vi "MainTemplate.vi"() -> ()   [LabVIEW 2017]
uses:
  <vilib>/Utility/cursorutil.llb/Set Cursor (Icon Pict).vi
panel:
  out "Admin?":bool
  out "DAQmx":tag
  in  "EventTimeout":i32=100
  out "TestArray":string[](array[string])
  out "PN":string
  out "FileName":string
  out "UUT SoftwareVer":string
  out "SN From File":string
  out "ProductRev":string
  out "UUT In":u16(ring)=4 items=["BLDC  60A  P/N: 1"=1, "BLDC  30A  P/N: 2"=2, "Warrior 60A P/N: 3"=3, "Condenser Merkava P/N: 4"=4, "Condenser India P/N: 4"=5]
  out "G.Stop":bool
  out "STDBY":bool
  out "TestinExecution":string
  out "User":string
  out "ParamVersion":string
  out "TesterVersion":string
  out "ClosePanel":bool=TRUE
  out "Automation":bool
  out "Test Failed":bool
  out "Next SN":i32
  in  "SetSN":bool
  out "UUT":u8
  out "UUT":string="EBAY"
  in  "Report":bool
  in  "Start":bool
  in  "ATR":string[][](table)=[["Test Communication", "-", "-", "-", "-", ""], ["Set S/N", "-", "-", "-", "-", ""], ["Set Board Number", "-", "-", "-", "-", ""], [" ", "", "", "", "", ""], ["Test Communication", "-", "-", "-", "-", ""], ["Get S/N", "-", "-", "-", "", ""], ["Get Board Number", "-", "-", "-", "", ""], ["Get FW", "-", "-", "-", "", ""], ["Enable Motor", "", "", "", "", ""], ["Small position command", "", "", "", "", ""], ["Measure delta", "", "", "", "", ""], ["Velocity command", "", "", "", "", ""]]
  in  "Settings":bool
  in  "Refresh Button":bool
  in  "VISA":refnum<visa-resource-name>="COM6"
  in  "Help Button":bool
  out "Pannel User Message":string
  in  "Stop Button":bool
  # "Template"
  # "REDLER TECHNOLOGIES LTD"
  # "ver 1.2p"
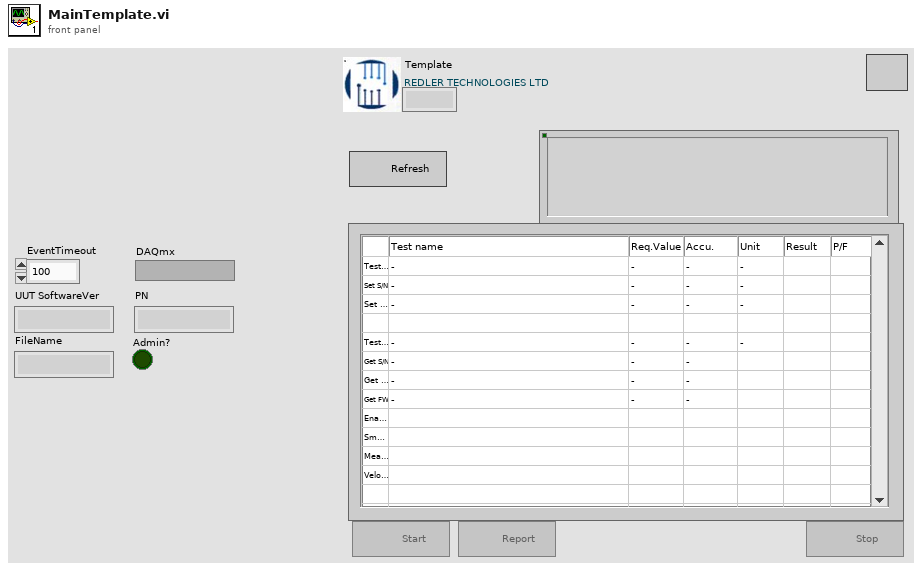
[diagram p1: front panel]
types:
  T1 = cluster{"VISA":refnum<visa-resource-name>, "TestArray":string[]}
  T2 = enum16{"Erase ATR Table", "Stop", "MainProgram", "Initialize"}
  T3 = enum8{"Enabled", "Disabled", "Disabled and Grayed Out"}
  T4 = enum32{"Invalid", "Standard", "Closed", "Hidden", "Minimized", "Maximized"}
  T5 = typedef "LVPoint32TypeDef.ctl" = cluster{"Horizontal":i32, "Vertical":i32}
  T6 = typedef "LVRowAndColumnTypeDef.ctl" = cluster{"Row":i32, "Column":i32}
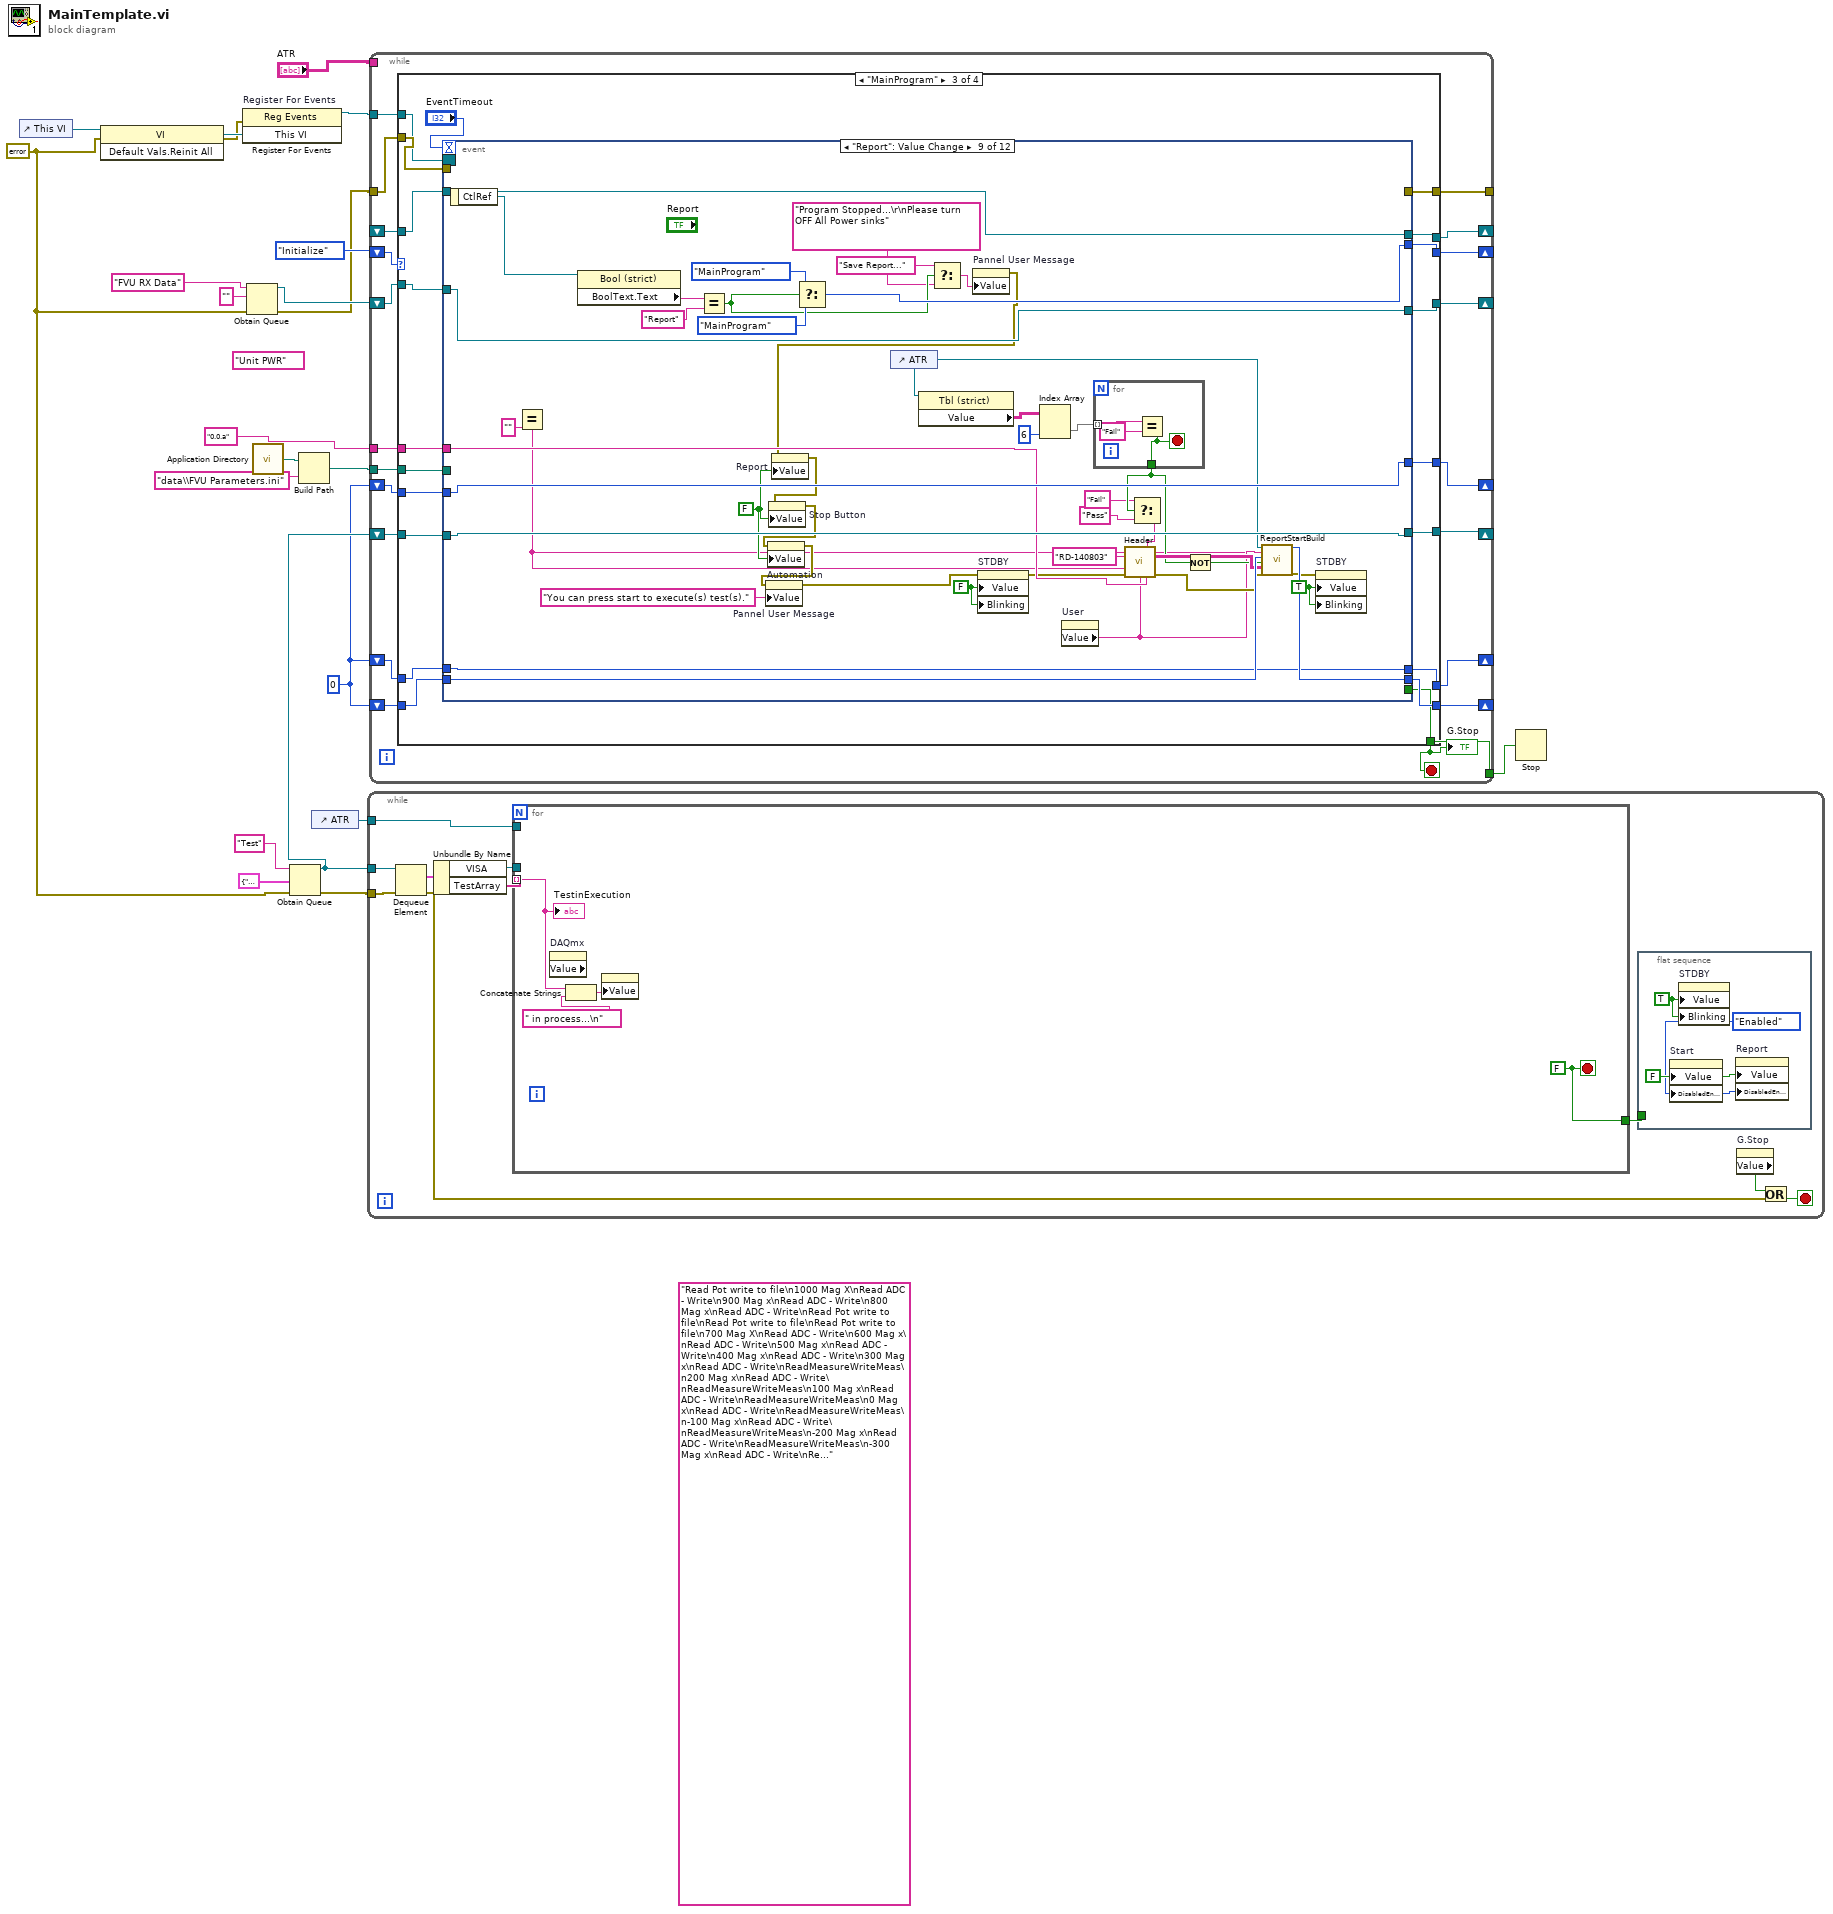
[diagram p0: block diagram]
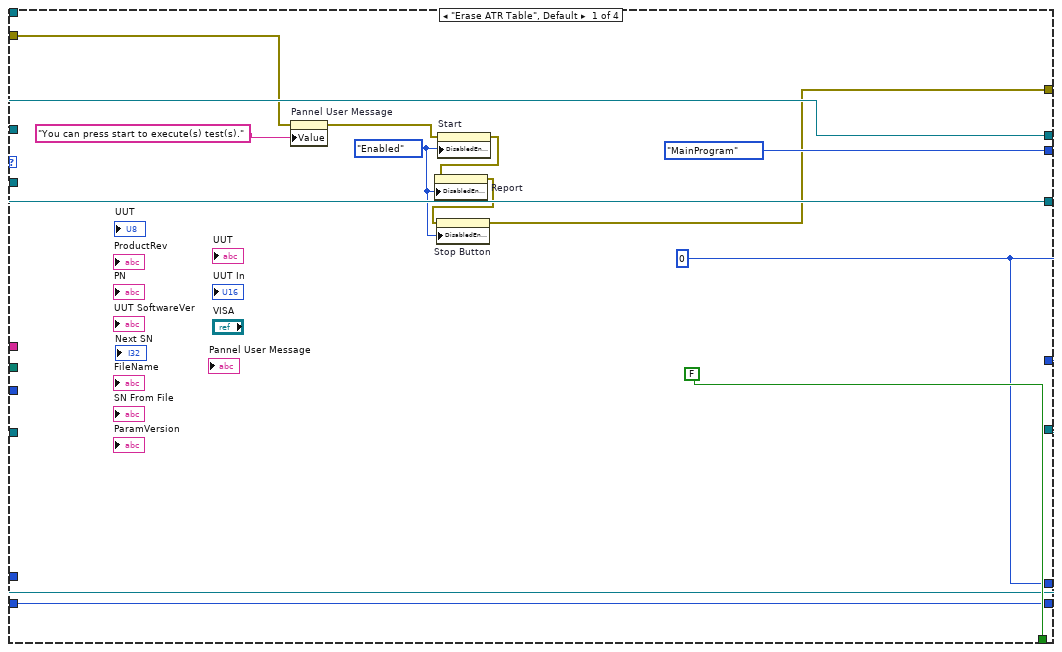
[diagram p2: hidden frame]
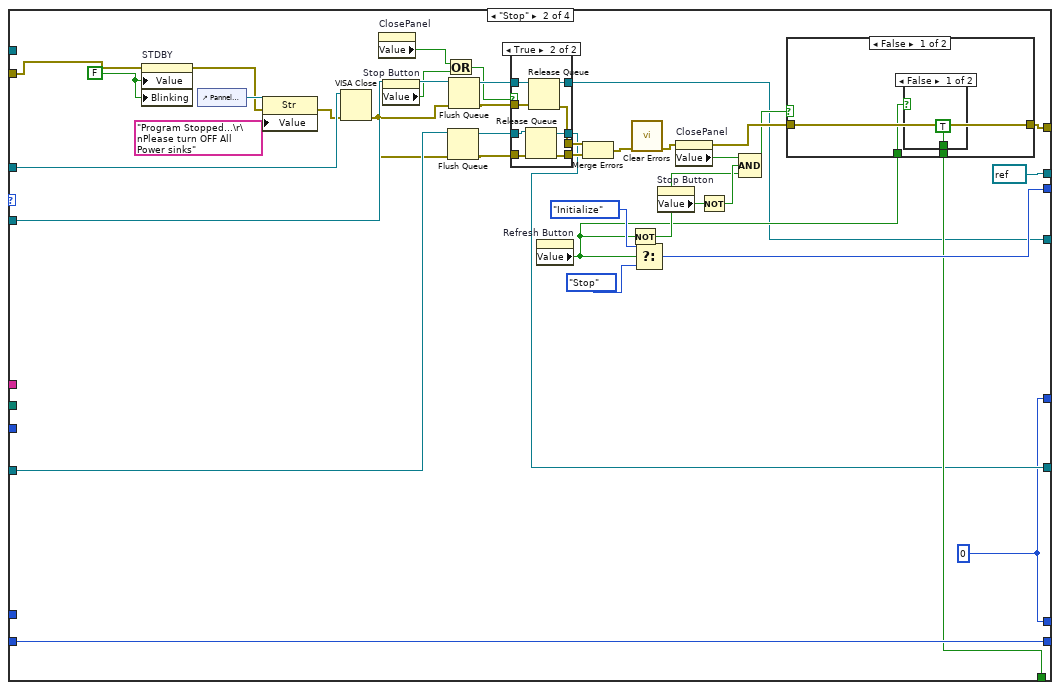
[diagram p3: hidden frame]
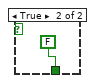
[diagram p5: hidden frame]
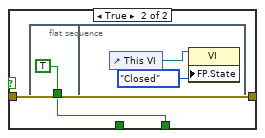
[diagram p6: hidden frame]
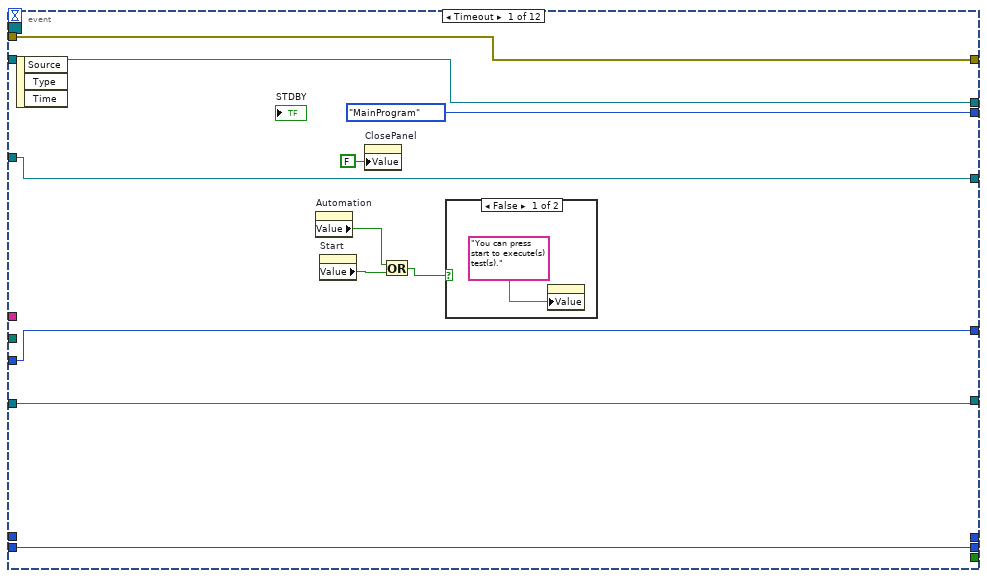
[diagram p7: hidden frame]
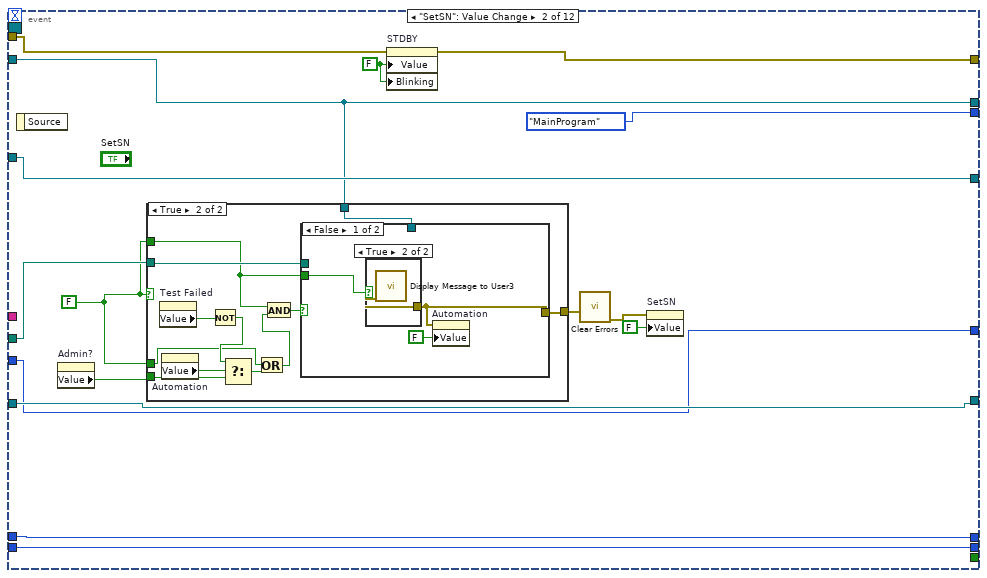
[diagram p9: hidden frame]
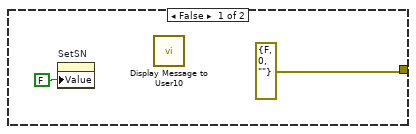
[diagram p10: hidden frame]
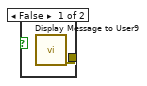
[diagram p11: hidden frame]
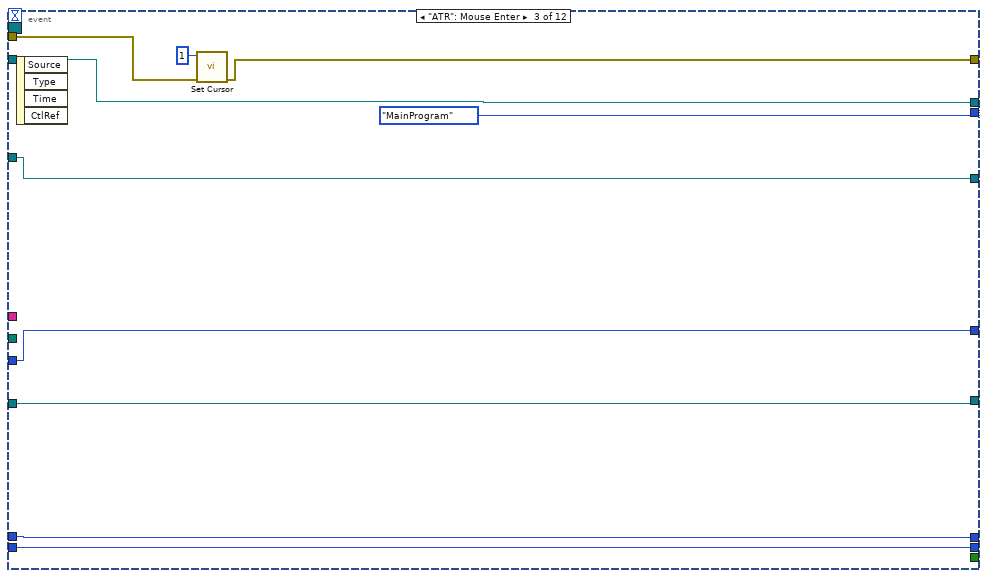
[diagram p13: hidden frame]
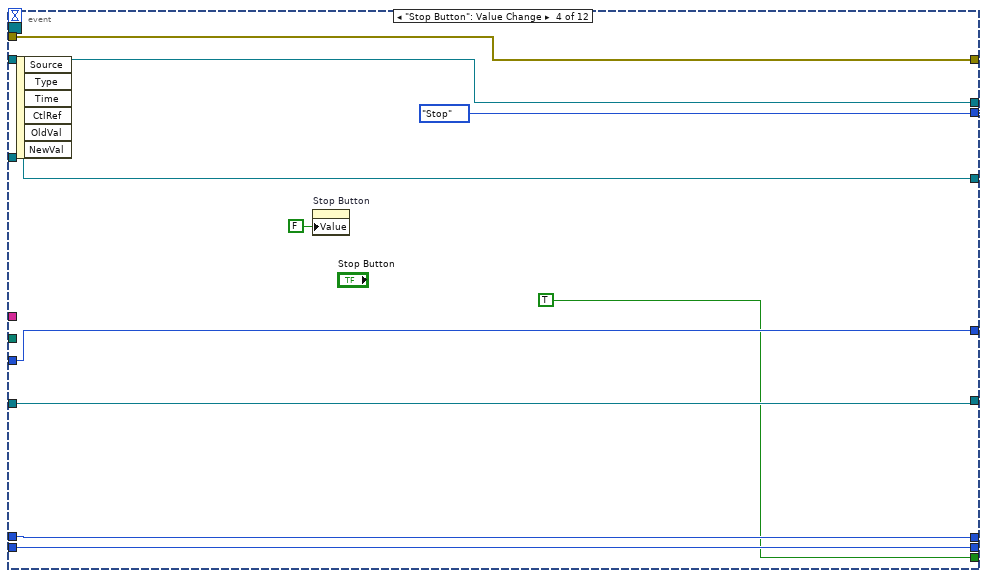
[diagram p14: hidden frame]
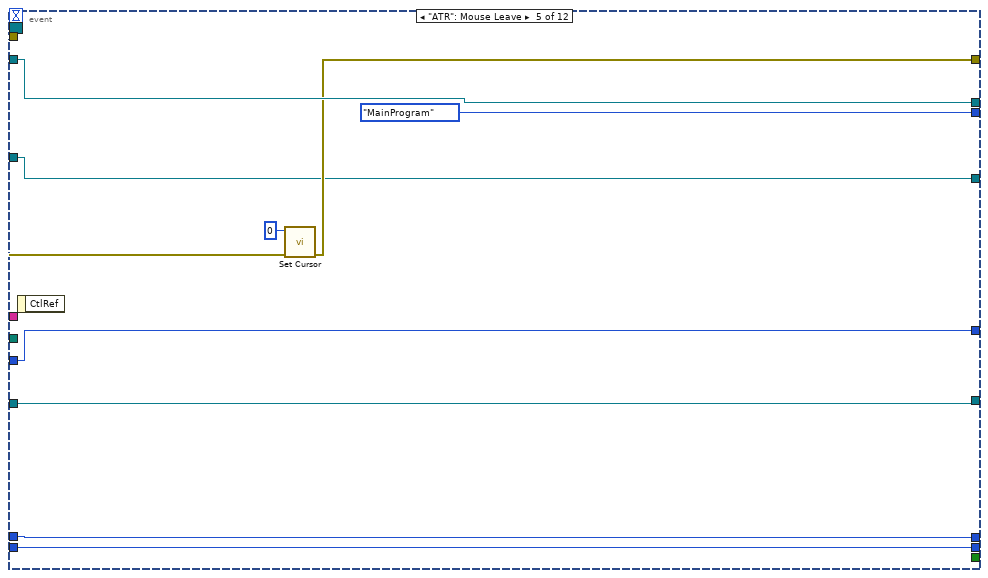
[diagram p15: hidden frame]
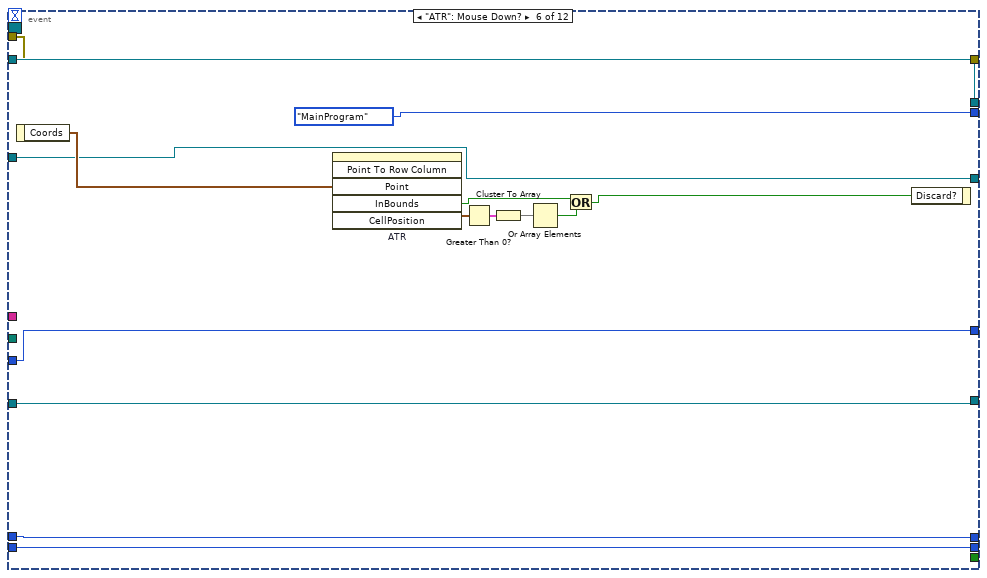
[diagram p16: hidden frame]
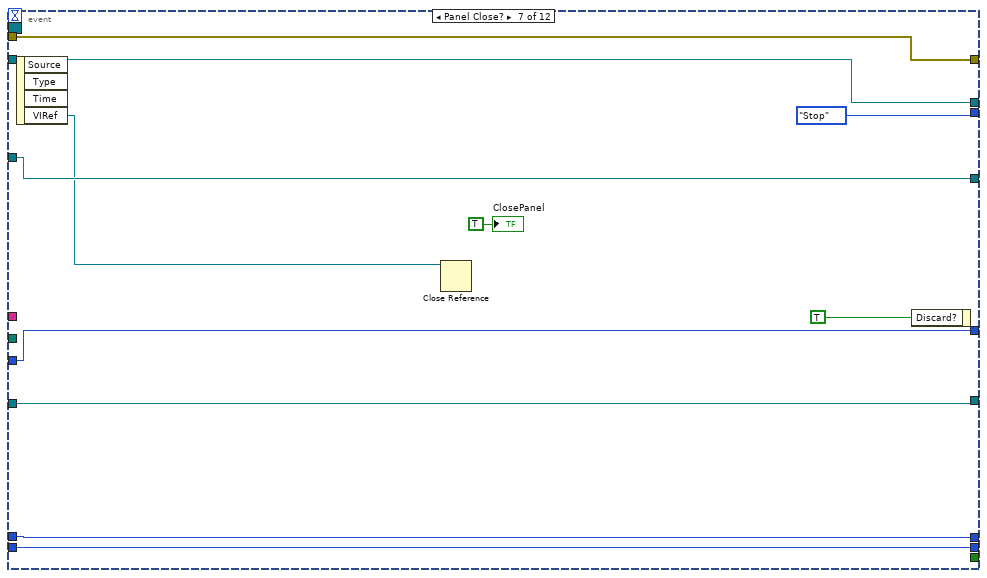
[diagram p17: hidden frame]
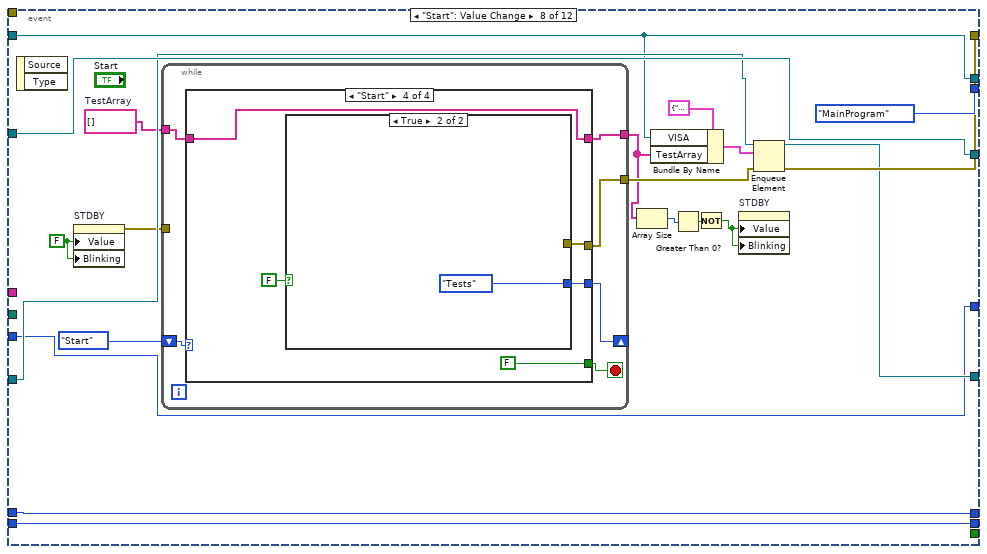
[diagram p18: hidden frame]
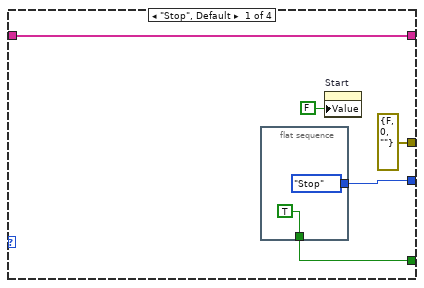
[diagram p19: hidden frame]
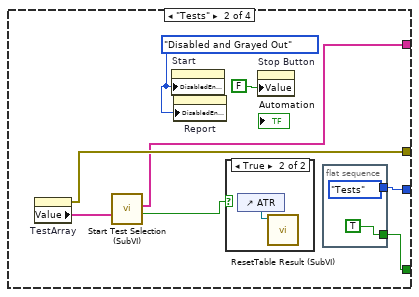
[diagram p20: hidden frame]
diagram:
  (unwired) "Read Pot write to file\n1000 Mag X\nRead ADC - Write\n900 Mag x\nRead ADC - Write\n800 Mag x\nRead ADC - Write\nRead Pot write to file\nRead Pot write to file\nRead Pot write to file\n700 Mag X\nRead ADC - Write\n600 Mag x\nRead ADC - Write\n500 Mag x\nRead ADC - Write\n400 Mag x\nRead ADC - Write\n300 Mag x\nRead ADC - Write\nReadMeasureWriteMeas\n200 Mag x\nRead ADC - Write\nReadMeasureWriteMeas\n100 Mag x\nRead ADC - Write\nReadMeasureWriteMeas\n0 Mag x\nRead ADC - Write\nReadMeasureWriteMeas\n-100 Mag x\nRead ADC - Write\nReadMeasureWriteMeas\n-200 Mag x\nRead ADC - Write\nReadMeasureWriteMeas\n-300 Mag x\nRead ADC - Write\nReadMeasureWriteMeas\n-400 Mag x\nRead ADC - Write\n-500 Mag x\nRead ADC - Write\n-600 Mag x\nRead ADC - Write\nRead Pot write to file\nRead Pot write to file\nRead Pot write to file\n-700 Mag x\nRead ADC - Write\n-800 Mag x\nRead ADC - Write\n-900 Mag x\nRead ADC - Write\n-1000 Mag x\nRead ADC - Write"
  (unwired) "Unit PWR" ("Combo Box")
  w10 = 0
  w3 = errorcluster {"status"=FALSE, "code"=0, "source"=""} ("error in (no error)")
  n1 = control-ref of="This VI"() -> (w11:refnum<vi>)
  n2 = invoke class="VI" method="Default Vals.Reinit All"(reference=w11, error in=w3) -> (reference out=w6:refnum<vi>, error out=w1:errorcluster)  [unwired: 1 in, 1 out]
  n3 = register-events "Register For Events"(error in=w1, w6) -> (reference out=w13:refnum<event-registration>)  [unwired: 1 in, 1 out]
  n4 = Obtain Queue(name (unnamed)="FVU RX Data", element data type="", error in (no error)=w3) -> (queue out=w20:refnum<queue>, error out=w18:errorcluster)  [unwired: 2 in, 1 out]
  n5 = call <vilib>:"Application Directory.vi"() -> ("Application Directory"=w15:path)
  n6 = Obtain Queue(name (unnamed)="Test", element data type=T1 {"VISA"="COM1", "TestArray"=[]}, error in (no error)=w3) -> (queue out=w17:refnum<queue>, error out=w2:errorcluster)  [unwired: 2 in, 1 out]
  n7 = Build Path(base path=w15, name or relative path="data\\FVU Parameters.ini") -> (appended path=w7:path)
  n8 = control-ref of="ATR"() -> (w12:refnum<vi>)
  n9 = while {
    tunnel: w12 -> [w32]
    tunnel: w2 -> [w30]
    tunnel: w17 -> [w31]
    stop <- w24 stop-if-true
    n10 = Dequeue Element(queue=w31, error in (no error)=w30) -> (element=w29:T1, error out=w27:errorcluster)  [unwired: 1 in, 2 out]
    n11 = Unbundle By Name(w29) -> ("VISA"=w28:refnum<visa-resource-name>, "TestArray"=w25:string[])
    n12 = for {
      tunnel: w25 -> [w37] mode=indexing
      tunnel: w28 -> [_]
      tunnel: w32 -> [_]
      tunnel: [w39] -> w26
      stop <- w39 stop-if-true
      w39 = FALSE ("Stopped")
      n13 = property on="DAQmx" class="DAQmxName" props=["Value"]() -> ()  [unwired: 2 in, 3 out]
      n14 = Concatenate Strings(w37, " in process...\n" ("string")) -> (w36:string)
      n15 = property on="Pannel User Message" class="Str"("Value"=w36) -> ()  [unwired: 2 in, 2 out]
      "TestinExecution" <- w37
    }
    n16 = flat-sequence {
      tunnel: w26 -> [_]
      frame #0 {
        w33 = TRUE ("STDBY")
        w34 = T3."Enabled" ("Disabled")
        w35 = FALSE ("Start")
        n17 = property on="Start" class="Bool (strict)"("Value"=w35, "DisabledEnum"=w34) -> ()  [unwired: 2 in, 2 out]
        n18 = property on="STDBY" class="Bool (strict)"("Value"=w33, "Blinking"=w33) -> ()  [unwired: 2 in, 2 out]
        n19 = property on="Report" class="Bool (strict)"("Value"=w35, "DisabledEnum"=w34) -> ()  [unwired: 2 in, 2 out]
      }
    }
    n20 = property on="G.Stop" class="Bool (strict)"() -> ("Value"=w23:bool)  [unwired: 2 in, 2 out]
    n21 = Or(x=w23, y=w27) -> (x .or. y?=w24:bool)
  }
  n22 = while {
    shift-right: [w46] -> _
    shift-left: T2."Initialize" -> [w40]
    shift-right: [w57] -> _
    shift-left: _ -> [w56]
    shift-right: [w55] -> _
    shift-left: w20 -> [w54]
    shift-right: [w52] -> _
    shift-left: w17 -> [w53]
    tunnel: "ATR" -> [_]
    tunnel: w13 -> [w51]
    shift-right: [w49] -> _
    shift-left: w10 -> [w50]
    tunnel: w7 -> [w48]
    tunnel: w18 -> [w59]
    tunnel: [w58] -> _
    tunnel: "0.0.a" -> [w47]
    shift-right: [w44] -> _
    shift-left: w10 -> [w45]
    shift-right: [w42] -> _
    shift-left: w10 -> [w43]
    tunnel: [w41] -> w8
    stop <- w41 stop-if-true
    n23 = case shown="\"MainProgram\"" w40 {
      tunnel: [T2."MainProgram" w98 w151 T2."Erase ATR Table"] -> w46
      tunnel: [FALSE w87 w132 FALSE] -> w41
      tunnel: [w61 w91 w146 w395] -> w58
      tunnel: w59 -> [w60 w78 w150 w395]
      tunnel: [w63 refnum<visa-resource-name> refnum ("VISA resource name") w147 w392] -> w57
      tunnel: w56 -> [w63 w108 w148 _]
      tunnel: [w72 w81 w144 w398] -> w55
      tunnel: w54 -> [w72 w110 w145 w398]
      tunnel: w53 -> [w71 w104 w143 w397]
      tunnel: [w71 w80 w142 w397] -> w52
      tunnel: w51 -> [_ _ w141 _]
      tunnel: w50 -> [w70 w102 w140 w396]
      tunnel: [w70 w102 w139 w396] -> w49
      tunnel: w48 -> [_ _ w138 _]
      tunnel: w47 -> [_ _ w137 w391]
      tunnel: w45 -> [_ _ w136 _]
      tunnel: [w69 w79 w135 w394] -> w44
      tunnel: w43 -> [_ _ w134 _]
      tunnel: [w69 w79 w133 w394] -> w42
      frame "Erase ATR Table", Default {
        w69 = 0
        w64 = T3."Enabled" ("Disabled")
        n24 = property on="Pannel User Message" class="Str"(error in=w60, "Value"="You can press start to execute(s) test(s)." ("Pannel User Message")) -> (error out=w62:errorcluster)  [unwired: 1 in, 1 out]
        n25 = property on="Start" class="Bool (strict)"(error in=w62, "DisabledEnum"=w64) -> (error out=w67:errorcluster)  [unwired: 1 in, 1 out]
        n26 = property on="Report" class="Bool (strict)"(error in=w67, "DisabledEnum"=w64) -> (error out=w65:errorcluster)  [unwired: 1 in, 1 out]
        n27 = property on="Stop Button" class="Bool (strict)"(error in=w65, "DisabledEnum"=w64) -> (error out=w61:errorcluster)  [unwired: 1 in, 1 out]
      }
      frame "Stop" {
        w77 = FALSE ("STDBY")
        w79 = 0
        n28 = property on="STDBY" class="Bool (strict)"(error in=w78, "Value"=w77, "Blinking"=w77) -> (error out=w74:errorcluster)  [unwired: 1 in, 1 out]
        n29 = control-ref of="Pannel User Message"() -> (w76:refnum<vi>)
        n30 = property class="Str"(reference=w76, error in=w74, "Value"="Program Stopped...\r\nPlease turn OFF All Power sinks") -> (error out=w101:errorcluster)  [unwired: 1 out]
        n31 = VISA Close(VISA resource name=w108, error in (no error)=w101) -> (error out=w103:errorcluster)
        n32 = property on="ClosePanel" class="Bool (strict)"() -> ("Value"=w84:bool)  [unwired: 2 in, 2 out]
        n33 = property on="Stop Button" class="Bool (strict)"() -> ("Value"=w83:bool)  [unwired: 2 in, 2 out]
        n34 = Or(x=w84, y=w83) -> (x .or. y?=w82:bool)
        n35 = Flush Queue(queue=w104, error in (no error)=w103) -> (queue out=w106:refnum<queue>, error out=w105:errorcluster)  [unwired: 1 out]
        n36 = Flush Queue(queue=w110, error in (no error)=w103) -> (queue out=w109:refnum<queue>, error out=w111:errorcluster)  [unwired: 1 out]
        n37 = case shown="True" w82 {
          tunnel: w111 -> [w113 w121]
          tunnel: w109 -> [w115 w117]
          tunnel: w106 -> [w114 w116]
          tunnel: w105 -> [w112 w120]
          tunnel: [w113 w119] -> w97
          tunnel: [w112 w118] -> w96
          tunnel: [w115 w117] -> w81
          tunnel: [w114 w116] -> w80
          frame False {
          }
          frame True {
            n38 = Release Queue(queue=w116, error in (no error)=w120) -> (error out=w118:errorcluster)  [unwired: 1 in, 2 out]
            n39 = Release Queue(queue=w117, error in (no error)=w121) -> (error out=w119:errorcluster)  [unwired: 1 in, 2 out]
          }
        }
        n40 = property on="Refresh Button" class="Bool (strict)"() -> ("Value"=w85:bool)  [unwired: 2 in, 2 out]
        n41 = Merge Errors(w97, w96) -> (w95:errorcluster)
        n42 = Not(x=w85) -> (.not. x?=w86:bool)
        n43 = call <vilib>:"Clear Errors.vi"("error in (no error)"=w95) -> ("error out"=w94:errorcluster)  [unwired: 5 in, 1 out]
        n44 = Select(t=T2."Initialize", s=w85, f=T2."Stop") -> (s? t:f=w98:T2)
        n45 = property on="Stop Button" class="Bool (strict)"() -> ("Value"=w89:bool)  [unwired: 2 in, 2 out]
        n46 = property on="ClosePanel" class="Bool (strict)"(error in=w94) -> (error out=w92:errorcluster, "Value"=w93:bool)  [unwired: 1 in, 1 out]
        n47 = Not(x=w89) -> (.not. x?=w88:bool)
        n48 = Compound Arithmetic op=AND(w93, w88, w86) -> (w90:bool)
        n49 = case shown="False" w90 {
          tunnel: w92 -> [w124 w128]
          tunnel: [w124 w128] -> w91
          tunnel: [w123 w127] -> w87
          tunnel: w85 -> [w122 _]
          frame False {
            n50 = case shown="False" w122 {
              tunnel: [TRUE FALSE] -> w123
              frame False {
              }
              frame True {
              }
            }
          }
          frame True {
            n51 = flat-sequence {
              tunnel: [TRUE] -> w127
              frame #0 {
              }
              frame #1 {
                n52 = control-ref of="This VI"() -> (w131:refnum<vi>)
                n53 = property class="VI"(reference=w131, "FP.State"=T4."Closed" ("Front Panel Window:State")) -> ()  [unwired: 1 in, 2 out]
              }
            }
          }
        }
      }
      frame "MainProgram" {
        n54 = event shown="[8] \"Report\": Value Change" {
          selector: w141 -> [_ _ _ _ _ _ _ _ _ _ _ _]
          dyn-events: _ -> [_ _ _ _ _ _ _ _ _ _ _ _]
          timeout: "EventTimeout" -> [_ _ _ _ _ _ _ _ _ _ _ _]
          tunnel: [T2."MainProgram" T2."MainProgram" T2."MainProgram" T2."Stop" T2."MainProgram" T2."MainProgram" T2."Stop" T2."MainProgram" w346 T2."MainProgram" T2."Stop" T2."MainProgram"] -> w151
          tunnel: [w158 w165 w207 w217 w225 w235 w254 w271 w339 w370 w382 w383] -> w146
          tunnel: w150 -> [w158 w168 w206 w217 w227 w235 w254 _ w339 w359 w382 w383]
          tunnel: [w156 w174 w208 w218 w226 w236 w252 w264 w312 w368 w380 w386] -> w147
          tunnel: w148 -> [w156 w174 w208 w218 w226 w236 w252 w264 w312 w368 w380 w386]
          tunnel: w145 -> [w161 w179 w203 w215 w223 w233 w251 w273 w354 w367 w379 w389]
          tunnel: [w161 w179 w203 w215 w223 w233 w251 w273 w354 w367 w379 w389] -> w144
          tunnel: w143 -> [w155 w178 w202 w214 w222 w232 w250 w272 w353 w366 w378 w388]
          tunnel: [w155 w178 w202 w214 w222 w232 w250 w270 w353 w366 w378 w388] -> w142
          tunnel: w140 -> [w160 w177 w201 w213 w221 w231 w248 w268 w352 w365 w377 w387]
          tunnel: [w160 w177 w201 w213 w221 w231 w248 w268 w351 w365 w377 w387] -> w139
          tunnel: w138 -> [_ w175 _ _ _ _ _ _ _ _ _ _]
          tunnel: w137 -> [_ _ _ _ _ _ _ _ w333 w364 _ _]
          tunnel: w136 -> [_ w170 w200 w212 w220 w230 w245 w267 w340 w362 w376 w385]
          tunnel: [_ w170 w200 w212 w220 w230 w245 w267 w340 w362 w376 w385] -> w135
          tunnel: w134 -> [w157 w169 w199 w211 w219 w229 w244 w266 w337 w361 w375 w384]
          tunnel: [w157 w169 w199 w211 w219 w229 w244 w266 w337 w361 w375 w384] -> w133
          tunnel: [_ _ _ TRUE _ _ _ _ _ _ _ _] -> w132
          event Timeout {
            n55 = event-data() -> ()  [unwired: 1 in, 3 out]
            n56 = property on="Automation" class="Bool (strict)"() -> ("Value"=w154:bool)  [unwired: 2 in, 2 out]
            n57 = property on="Start" class="Bool (strict)"() -> ("Value"=w152:bool)  [unwired: 2 in, 2 out]
            n58 = property on="ClosePanel" class="Bool (strict)"("Value"=FALSE ("ClosePanel")) -> ()  [unwired: 2 in, 2 out]
            n59 = Or(x=w154, y=w152) -> (x .or. y?=w153:bool)
            n60 = case shown="False" w153 {
              frame False {
                n61 = property on="Pannel User Message" class="Str"("Value"="You can press start to execute(s) test(s).") -> ()  [unwired: 2 in, 2 out]
              }
              frame True {
              }
            }
          }
          event "SetSN": Value Change {
            w164 = FALSE ("Value")
            w167 = FALSE ("STDBY")
            n62 = event-data() -> ()  [unwired: 1 in, 1 out]
            n63 = property on="Admin?" class="Bool (strict)"() -> ("Value"=w166:bool)  [unwired: 2 in, 2 out]
            n64 = case shown="True" w164 {
              tunnel: w175 -> [_ w193]
              tunnel: w164 -> [_ w182]
              tunnel: w174 -> [_ w192]
              tunnel: w166 -> [_ w191]
              tunnel: [errorcluster {"status"=FALSE, "code"=0, "source"=""} ("error out") w190] -> w173
              tunnel: w164 -> [_ w183]
              frame False {
                n65 = property on="SetSN" class="Bool (strict)"("Value"=FALSE) -> ()  [unwired: 2 in, 2 out]
                n66 = call "Display Message to User10"() -> ()  [unwired: 10 in, 2 out]
              }
              frame True {
                n67 = property on="Test Failed" class="Bool (strict)"() -> ("Value"=w187:bool)  [unwired: 2 in, 2 out]
                n68 = property on="Automation" class="Bool (strict)"() -> ("Value"=w189:bool)  [unwired: 2 in, 2 out]
                n69 = Not(x=w187) -> (.not. x?=w188:bool)
                n70 = Select(t=w188, s=w189, f=w191) -> (s? t:f=w185:bool)
                n71 = Or(x=w183, y=w185) -> (x .or. y?=w184:bool)
                n72 = And(x=w182, y=w184) -> (x .and. y?=w186:bool)
                n73 = case shown="False" w186 {
                  tunnel: w193 -> [_ _]
                  tunnel: w192 -> [_ _]
                  tunnel: [w195 _] -> w190
                  tunnel: w182 -> [w194 _]
                  frame False {
                    n74 = case shown="True" w194 {
                      tunnel: [w197 w198] -> w195
                      frame False {
                        n75 = call "Display Message to User9"() -> ("error out"=w197:errorcluster)  [unwired: 10 in, 1 out]
                      }
                      frame True {
                        n76 = call "Display Message to User3"() -> ("error out"=w198:errorcluster)  [unwired: 10 in, 1 out]
                      }
                    }
                    n77 = property on="Automation" class="Bool (strict)"(error in=w195, "Value"=FALSE ("Automation")) -> ()  [unwired: 1 in, 2 out]
                  }
                  frame True {
                  }
                }
              }
            }
            n78 = property on="STDBY" class="Bool (strict)"(error in=w168, "Value"=w167, "Blinking"=w167) -> (error out=w165:errorcluster)  [unwired: 1 in, 1 out]
            n79 = call <vilib>:"Clear Errors.vi"("error in (no error)"=w173) -> ("error out"=w171:errorcluster)  [unwired: 5 in, 1 out]
            n80 = property on="SetSN" class="Bool (strict)"(error in=w171, "Value"=FALSE ("SetSN")) -> ()  [unwired: 1 in, 2 out]
          }
          event "ATR": Mouse Enter {
            n81 = event-data() -> ()  [unwired: 1 in, 4 out]
            n82 = call-poly <vilib>:"Set Cursor.vi"("error in (no error)"=w206, "icon"=u16 1) -> ("error out"=w207:errorcluster)  [unwired: 8 in, 1 out]
          }
          event "Stop Button": Value Change {
            n83 = event-data() -> ()  [unwired: 1 in, 6 out]
            n84 = property on="Stop Button" class="Bool (strict)"("Value"=FALSE ("Stop Button")) -> ()  [unwired: 2 in, 2 out]
          }
          event "ATR": Mouse Leave {
            n85 = event-data() -> ()  [unwired: 1 in, 1 out]
            n86 = call-poly <vilib>:"Set Cursor.vi"("error in (no error)"=w227, "icon"=u16 0) -> ("error out"=w225:errorcluster)  [unwired: 8 in, 1 out]
          }
          event "ATR": Mouse Down? {
            n87 = event-data() -> ("Coords"=w243:T5)  [unwired: 1 in]
            n88 = invoke on="ATR" class="Tbl (strict)" method="Point To Row Column"("Point"=w243) -> ("InBounds"=w239:bool, "CellPosition"=w238:T6)  [unwired: 5 in, 4 out]
            n89 = Greater Than 0?(x=w238) -> (x > 0?=w242:cluster{"Row":bool, "Column":bool})
            n90 = Cluster To Array(cluster=w242) -> (array=w241:bool[])
            n91 = Or Array Elements(Boolean array=w241) -> (logical OR=w240:bool)
            n92 = Or(x=w239, y=w240) -> (x .or. y?=w237:bool)
            n93 = event-data("Discard?"=w237) -> ()  [unwired: 1 in, 1 out]
          }
          event Panel Close? {
            n94 = event-data() -> ("VIRef"=w249:refnum<vi>)  [unwired: 1 in, 3 out]
            n95 = Close Reference(reference=w249) -> ()  [unwired: 1 in, 1 out]
            n96 = event-data("Discard?"=TRUE) -> ()  [unwired: 1 in, 1 out]
            "ClosePanel" <- TRUE ("ClosePanel")
          }
          event "Start": Value Change {
            w260 = FALSE ("STDBY")
            w262 = string[] []  # TestArray
            n97 = event-data() -> ()  [unwired: 1 in, 2 out]
            n98 = property on="STDBY" class="Bool (strict)"("Value"=w260, "Blinking"=w260) -> (error out=w261:errorcluster)  [unwired: 2 in, 1 out]
            n99 = while {
              tunnel: [w280] -> w258
              tunnel: [w279] -> w259
              shift-right: [w277] -> _
              shift-left: enum16{"Stop", "Tests", "Bit test", "Start"}."Start" -> [w278]
              tunnel: w262 -> [w276]
              tunnel: w261 -> [_]
              stop <- w275 stop-if-true
              n100 = case shown="\"Start\"" w278 {
                tunnel: [w285 w288 w299 w307] -> w280
                tunnel: [errorcluster {"status"=FALSE, "code"=0, "source"=""} ("error out") w291 errorcluster {"status"=FALSE, "code"=0, "source"=""} ("error out") w305] -> w279
                tunnel: [w284 w295 enum16{"Stop", "Tests", "Bit test", "Start"}."Stop" w304] -> w277
                tunnel: w276 -> [w285 _ w299 w307]
                tunnel: [w283 w294 FALSE FALSE] -> w275
                frame "Stop", Default {
                  n101 = flat-sequence {
                    tunnel: [enum16{"Stop", "Tests", "Bit test", "Start"}."Stop"] -> w284
                    tunnel: [TRUE] -> w283
                    frame #0 {
                    }
                  }
                  n102 = property on="Start" class="Bool (strict)"("Value"=FALSE ("Start")) -> ()  [unwired: 2 in, 2 out]
                }
                frame "Tests" {
                  w293 = T3."Disabled and Grayed Out" ("Disabled")
                  n103 = property on="TestArray" class="Arr (strict)"() -> (error out=w291:errorcluster, "Value"=w290:string[])  [unwired: 2 in, 1 out]
                  n104 = call "Start Test Selection (SubVI).vi"("TestArrayIn"=w290) -> ("AutoOut"=w289:bool, "TestArrayOut"=w288:string[])  [unwired: 9 in]
                  n105 = property on="Start" class="Bool (strict)"("DisabledEnum"=w293) -> ()  [unwired: 2 in, 2 out]
                  n106 = property on="Report" class="Bool (strict)"("DisabledEnum"=w293) -> ()  [unwired: 2 in, 2 out]
                  n107 = case shown="True" w289 {
                    frame False {
                    }
                    frame True {
                      n108 = control-ref of="ATR"() -> (w296:refnum<vi>)
                      n109 = call "ResetTable Result (SubVI).vi"("Table in"=w296) -> ()  [unwired: 11 in]
                    }
                  }
                  n110 = property on="Stop Button" class="Bool (strict)"("Value"=FALSE ("Stop Burn-in")) -> ()  [unwired: 2 in, 2 out]
                  n111 = flat-sequence {
                    tunnel: [enum16{"Stop", "Tests", "Bit test", "Start"}."Tests"] -> w295
                    tunnel: [TRUE] -> w294
                    frame #0 {
                    }
                  }
                }
                frame "Bit test" {
                }
                frame "Start" {
                  n112 = case shown="True" FALSE {
                    tunnel: [w309 _] -> w305
                    tunnel: [enum16{"Stop", "Tests", "Bit test", "Start"}."Stop" enum16{"Stop", "Tests", "Bit test", "Start"}."Tests"] -> w304
                    frame False {
                      n113 = call "Display Message to User5"() -> ("error out"=w309:errorcluster)  [unwired: 10 in, 1 out]
                    }
                    frame True {
                    }
                  }
                }
              }
            }
            n114 = Array Size(array=w258) -> (size(s)=w257:i32)
            n115 = Bundle By Name(cluster=T1 {"VISA"="COM1", "TestArray"=[]}, "VISA"=w264, "TestArray"=w258) -> (w265:T1)
            n116 = Greater Than 0?(x=w257) -> (x > 0?=w256:bool)
            n117 = Not(x=w256) -> (.not. x?=w255:bool)
            n118 = property on="STDBY" class="Bool (strict)"("Value"=w255, "Blinking"=w255) -> ()  [unwired: 2 in, 2 out]
            n119 = Enqueue Element(queue=w272, element=w265, error in (no error)=w259) -> (queue out=w270:refnum<queue>, error out=w271:errorcluster)  [unwired: 2 out]
          }
          event "Report": Value Change {
            w311 = ""
            w316 = FALSE ("Report")
            w335 = TRUE ("STDBY")
            w338 = FALSE ("STDBY")
            n120 = event-data() -> ("CtlRef"=w350:refnum<vi>)  [unwired: 1 in]
            n121 = Equal?(x=w311, y=w311) -> ()  [unwired: 1 out]
            n122 = property class="Bool (strict)"(reference=w350) -> ("BoolText.Text"=w349:string)  [unwired: 1 in, 2 out]
            n123 = Equal?(x=w349, y="Report") -> (x = y?=w344:bool)
            n124 = Select(t=T2."MainProgram", s=w344, f=T2."MainProgram") -> (s? t:f=w346:T2)
            n125 = control-ref of="ATR"() -> (w331:refnum<vi>)
            n126 = property class="Tbl (strict)"(reference=w331) -> ("Value"=w330:string[][])  [unwired: 1 in, 2 out]
            n127 = Select(t="Save Report...", s=w344, f="Program Stopped...\r\nPlease turn OFF All Power sinks") -> (s? t:f=w342:string)
            n128 = property on="Pannel User Message" class="Str"("Value"=w342) -> (error out=w313:errorcluster)  [unwired: 2 in, 1 out]
            n129 = property on="Report" class="Bool (strict)"(error in=w313, "Value"=w316) -> (error out=w319:errorcluster)  [unwired: 1 in, 1 out]
            n130 = property on="Stop Button" class="Bool (strict)"(error in=w319, "Value"=w316) -> (error out=w318:errorcluster)  [unwired: 1 in, 1 out]
            n131 = property on="Automation" class="Bool (strict)"(error in=w318, "Value"=w316) -> (error out=w317:errorcluster)  [unwired: 1 in, 1 out]
            n132 = property on="Pannel User Message" class="Str"(error in=w317, "Value"="You can press start to execute(s) test(s)." ("Pannel User Message")) -> (error out=w314:errorcluster)  [unwired: 1 in, 1 out]
            n133 = property on="STDBY" class="Bool (strict)"(error in=w314, "Value"=w338, "Blinking"=w338) -> (error out=w322:errorcluster)  [unwired: 1 in, 1 out]
            n134 = Index Array(array=w330, index (col)=6 ("disabled index (col)")) -> (element=w328:string[])  [unwired: 1 in]
            n135 = property on="User" class="Str"() -> ("Value"=w320:string)  [unwired: 2 in, 2 out]
            n136 = for {
              tunnel: w328 -> [w357] mode=indexing
              tunnel: [w355] -> w327
              stop <- w355 stop-if-true
              n137 = Equal?(x=w357, y="Fail") -> (x = y?=w355:bool)
            }
            n138 = Select(t="Fail" ("y"), s=w327, f="Pass" ("y")) -> (s? t:f=w323:string)
            n139 = call "Header.vi"("GeneralResult"=w323, "P/N UUT"="RD-140803", "Driver S/N"=w311, "error in"=w322, "Oper."=w320, "Tester Software Ver"=w333) -> ("Array"=w336:string[][], "error out"=w321:errorcluster)  [unwired: 8 in]
            n140 = Not(x=w327) -> (.not. x?=w326:bool)
            n141 = call "ReportStartBuild.vi"("Table in"=w331, "Operator"=w320, "Numeric in"=w352, "GeneralResult-Pass(T)Fail(F)"=w326, "Header Array"=w336, "error in (no error)"=w321, "SN"=w311) -> ("Numeric out"=w351:i32, "error out"=w334:errorcluster)  [unwired: 11 in]
            n142 = property on="STDBY" class="Bool (strict)"(error in=w334, "Value"=w335, "Blinking"=w335) -> ()  [unwired: 1 in, 2 out]
          }
          event "Help Button": Value Change {
            w360 = FALSE ("STDBY")
            n143 = event-data() -> ()  [unwired: 1 in, 1 out]
            n144 = property on="STDBY" class="Bool (strict)"(error in=w359, "Value"=w360, "Blinking"=w360) -> (error out=w358:errorcluster)  [unwired: 1 in, 1 out]
            n145 = vi-ref "Help.vi"() -> (w372:refnum<vi>)
            n146 = invoke class="VI" method="FP.Open"(reference=w372, error in=w358, "Activate"=TRUE ("Activate?"), "State"=T4."Standard") -> (error out=w371:errorcluster)  [unwired: 1 in, 4 out]
            n147 = call "Help.vi"("error in"=w371, "TesterSWVersion"=w364) -> ("error out"=w370:errorcluster)  [unwired: 6 in]
            n148 = property on="Help Button" class="Bool (strict)"("Value"=FALSE ("Help Button")) -> ()  [unwired: 2 in, 2 out]
          }
          event "Refresh Button": Value Change {
            n149 = event-data() -> ()  [unwired: 1 in, 1 out]
          }
          event "Settings": Value Change {
            n150 = event-data() -> ()  [unwired: 1 in, 1 out]
          }
        }
      }
      frame "Initialize" {
        w394 = 0
        n151 = stacked-sequence {
          seq-local: [_ _ _ w433 _ _] -> [_ _ _ _ _ _]
          seq-local: [_ _ _ w431 _ _] -> [_ _ _ _ _ _]
          seq-local: [_ _ _ w430 _ _] -> [_ _ _ _ _ _]
          tunnel: [_ _ _ w433 _ _] -> w392
          frame #0 {
            w403 = FALSE ("STDBY")
            w405 = T3."Disabled and Grayed Out" ("Disabled")
            n152 = property on="Refresh Button" class="Bool (strict)"("Value"=FALSE ("Refresh Button")) -> ()  [unwired: 2 in, 2 out]
            n153 = property on="VISA" class="VISAName"("Visible"=FALSE, "Value"=refnum<visa-resource-name> "COMx" ("VISA Kinetics")) -> ()  [unwired: 2 in, 2 out]
            n154 = property on="Pannel User Message" class="Str"("Value"="Initialization State...") -> ()  [unwired: 2 in, 2 out]
            n155 = property on="Stop Button" class="Bool (strict)"("DisabledEnum"=w405) -> (error out=w407:errorcluster)  [unwired: 2 in, 1 out]
            n156 = property on="STDBY" class="Bool (strict)"("Value"=w403, "Blinking"=w403) -> ()  [unwired: 2 in, 2 out]
            n157 = property on="Start" class="Bool (strict)"(error in=w407, "DisabledEnum"=w405) -> (error out=w406:errorcluster)  [unwired: 1 in, 1 out]
            n158 = property on="Report" class="Bool (strict)"(error in=w406, "DisabledEnum"=w405) -> ()  [unwired: 1 in, 2 out]
            "Test Failed" <- FALSE ("Test Failed")
          }
          frame #1 {
            n159 = Two Button Dialog(message="Please choose ATP Mode", 1:"ESS" ("F button name (\"Cancel\")"), 2:"Normal" ("T button name (\"OK\")")) -> (T button?=w412:bool)
            n160 = control-ref of="ATR"() -> (w417:refnum<vi>)
            n161 = Select(t="data\\FVU_ATP.xlsx" ("name or relative path"), s=w412, f="data\\FVU_ATP_ESS.xlsx" ("name or relative path")) -> (s? t:f=w409:string)
            n162 = call "Init ATR Pannel from Excel (SubVI).vi"("name or relative path"=w409, "Table in"=w417) -> ("TestArray"=→"TestArray":string[])  [unwired: 9 in]
          }
          frame #2 {
            n163 = while {
              tunnel: [w426] -> _
              tunnel: [w419] -> _
              tunnel: [w424] -> w418
              stop <- w426 stop-if-true
              n164 = call "Operator Name"() -> ("Operator Name"=w419:string, "OK"=w427:bool)  [unwired: 17 in, 1 out]
              "User" <- w419
              n165 = To Lower Case(string=w419) -> (all lower case string=w420:string)
              n166 = Not Equal?(x=w419, y="") -> (x != y?=w428:bool)
              n167 = Equal?(x="Nisim", y=w419) -> (x = y?=w422:bool)
              n168 = Equal?(x="admin", y=w420) -> (x = y?=w425:bool)
              n169 = property on="User" class="Str"("Value"=w419) -> ()  [unwired: 2 in, 2 out]
              n170 = And(x=w427, y=w428) -> (x .and. y?=w426:bool)
              n171 = Or(x=w422, y=w425) -> (x .or. y?=w424:bool)
            }
            "Admin?" <- w418
          }
          frame #3 {
            n172 = call "Connect COM Port (SubVI).vi"() -> ("error out"=w436:errorcluster, "NoCOM PORT"=w430:bool, "VISA Refnum out"=w434:refnum<visa-resource-name>)  [unwired: 9 in]
            n173 = VISA Set I/O Buffer Size(VISA resource name=w434, size (4096)=u32 65535, error in (no error)=w436) -> (VISA resource name out=w433:refnum<visa-resource-name>, error out=w435:errorcluster)  [unwired: 1 in]
            n174 = call "Find DAQ Devices.vi"("Error In"=w435) -> ("DAQmx Device Name"=w431:tag)  [unwired: 8 in, 2 out]
            "DAQmx" <- w431
          }
          frame #4 {
          }
          frame #5 {
            w437 = TRUE ("STDBY")
            n175 = property on="STDBY" class="Bool (strict)"("Value"=w437, "Blinking"=w437) -> ()  [unwired: 2 in, 2 out]
          }
        }
        "TesterVersion" <- w391
      }
    }
    "G.Stop" <- w41
  }
  n176 = Stop(stop? (T)=w8) -> ()
